vi "DESTROY USER EVENTS.vi"(8 "error in (no error)":errorcluster, 11 "Measurement_Binary in":refnum<class "Measurement_Binary.lvclass">) -> (0 "error out":errorcluster, 3 "Measurement_Binary out":refnum<class "Measurement_Binary.lvclass">)   [LabVIEW 2020, in "Measurement_Binary.lvlib" / "Measurement_Binary.lvclass"]
uses:
  Measurement_Binary.lvclass
  Measurement_Binary.lvclass/Measurement_Binary.ctl
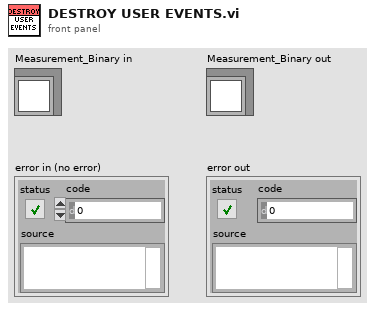
[diagram p1: front panel]
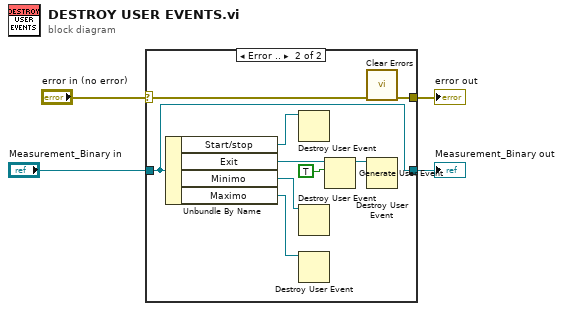
[diagram p0: block diagram]
diagram:
  n1 = case shown="Error .." "error in (no error)" {
    selector: "error in (no error)" -> [w5 w8]
    tunnel: "Measurement_Binary in" -> [w6 w15]
    tunnel: [w6 w15] -> w3
    tunnel: [w5 w7] -> w4
    frame No Error {
    }
    frame Error {
      n2 = Unbundle By Name(w15) -> ("Start/stop"=w11:refnum<user-event>, "Exit"=w14:refnum<user-event>, "Minimo"=w10:refnum<user-event>, "Maximo"=w9:refnum<user-event>)
      n3 = Destroy User Event(user event=w11) -> ()  [unwired: 1 in, 1 out]
      n4 = Destroy User Event(user event=w10) -> ()  [unwired: 1 in, 1 out]
      n5 = Destroy User Event(user event=w9) -> ()  [unwired: 1 in, 1 out]
      n6 = Generate User Event(user event=w14, event data cluster=TRUE ("event data")) -> (user event out=w12:refnum<user-event>)  [unwired: 2 in, 1 out]
      n7 = call <vilib>:"Clear Errors.vi"("error in (no error)"=w8) -> ("error out"=w7:errorcluster)  [unwired: 5 in, 1 out]
      n8 = Destroy User Event(user event=w12) -> ()  [unwired: 1 in, 1 out]
    }
  }
  "error out" <- w4
  "Measurement_Binary out" <- w3
